vi "RT PID.vi"(0 "setpoint":dbl, 1 "Encoder":i32, 3 "set PWM":bool, 4 "PWM value":i32, 5 "last error":dbl, 6 "gain_ff":cluster{"K_vff":dbl, "K_aff":dbl}, 7 "PID":cluster{"Kp":dbl, "Ki":dbl, "Kd":dbl}={"Kp"=5.0, "Ki"=0.0, "Kd"=300.0}, 9 "gain_ff":dbl, 10 "PWM Max":i32, 11 "V_ff":dbl, 13 "A_ff":dbl) -> (12 "P/D":cluster{dbl, dbl}, 14 "direction":bool, 15 "PD output":dbl, 16 "PWM value":dbl, 17 "ff output":dbl, 18 "PWM":i32, 19 "error":dbl)   [LabVIEW 2019]
panel:
  out "result":dbl
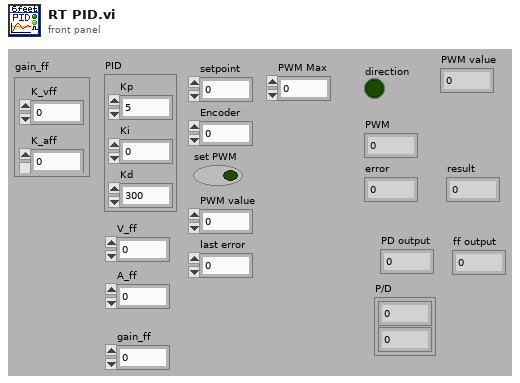
[diagram p1: front panel]
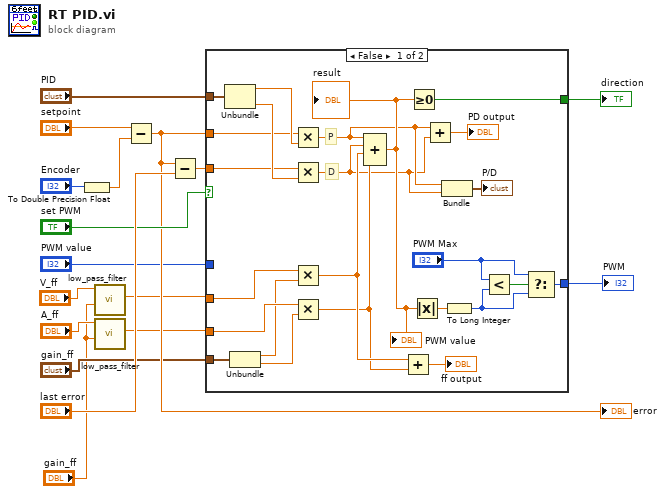
[diagram p0: block diagram]
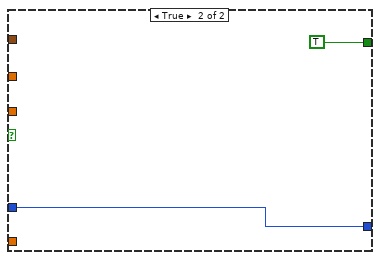
[diagram p2: hidden frame]
diagram:
  n1 = To Double Precision Float(number="Encoder") -> (double precision float=w9:dbl)
  n2 = call "low_pass_filter.vi"("gain"="gain_ff", "signal_now"="V_ff") -> ("filtered signal"=w4:dbl)  [unwired: 9 in]
  n3 = call "low_pass_filter.vi"("gain"="gain_ff", "signal_now"="A_ff") -> ("filtered signal"=w2:dbl)  [unwired: 9 in]
  n4 = Subtract(x="setpoint", y=w9) -> (x-y=w8:dbl)
  "error" <- w8
  n5 = Subtract(x=w8, y="last error") -> (x-y=w17:dbl)
  n6 = case shown="False" "set PWM" {
    tunnel: w17 -> [w36 _]
    tunnel: w8 -> [w35 _]
    tunnel: [w30 TRUE] -> w16
    tunnel: "PID" -> [w34 _]
    tunnel: [w33 w42] -> w12
    tunnel: "PWM value" -> [_ w42]
    tunnel: "gain_ff" -> [w29 _]
    tunnel: w4 -> [w28 _]
    tunnel: w2 -> [w27 _]
    frame False {
      # "D"
      # "P"
      n7 = Unbundle(w34) -> ("Kp"=w37:dbl, "Kd"=w38:dbl)  [unwired: 1 out]
      n8 = Unbundle(w29) -> ("K_vff"=w26:dbl, "K_aff"=w25:dbl)
      n9 = Multiply(x=w35, y=w37) -> (x*y=w20:dbl)
      n10 = Multiply(x=w36, y=w38) -> (x*y=w19:dbl)
      n11 = Multiply(x=w28, y=w26) -> (x*y=w23:dbl)
      n12 = Multiply(x=w27, y=w25) -> (x*y=w22:dbl)
      n13 = Compound Arithmetic op=ADD(w20, w19, w23, w22) -> (w40:dbl)
      "result" <- w40
      "PWM value" <- w40
      n14 = Add(x=w23, y=w22) -> (x+y=→"ff output":dbl)
      n15 = Greater Or Equal To 0?(x=w40) -> (x >= 0?=w30:bool)
      n16 = Absolute Value(x=w40) -> (abs(x)=w31:dbl)
      n17 = Add(x=w20, y=w19) -> (x+y=→"PD output":dbl)
      n18 = Bundle(w20, w19) -> (→"P/D":cluster{dbl, dbl})  [unwired: 1 in]
      n19 = To Long Integer(number=w31) -> (32bit integer=w41:i32)
      n20 = Less?(x="PWM Max", y=w41) -> (x < y?=w39:bool)
      n21 = Select(t="PWM Max", s=w39, f=w41) -> (s? t:f=w33:i32)
    }
    frame True {
    }
  }
  "direction" <- w16
  "PWM" <- w12
